vi "R1SBRControl_Status.vi"(7 "LabVIEW Web Service Request":refnum<class "Web Request.lvclass">) -> (0 "error out":errorcluster, 3 "SBRData":T1)   [LabVIEW 2016]
uses:
  <vilib>/wsapi/Web Request.lvclass
  R1Controls/R1SBR_Status.ctl
  R1Controls/R1SBR_SetParams.ctl
panel:
  # "Use the Web Service Request input terminal to call the VIs on the Web Services palette. Do not remove it from the connector pane unless you don't need access to the palette."
  # "Each additional control wired to the connector pane will be available as an input in the URL. To include an indicator in terminal-mode output (the default setting), it must also be wired to the connector pane."
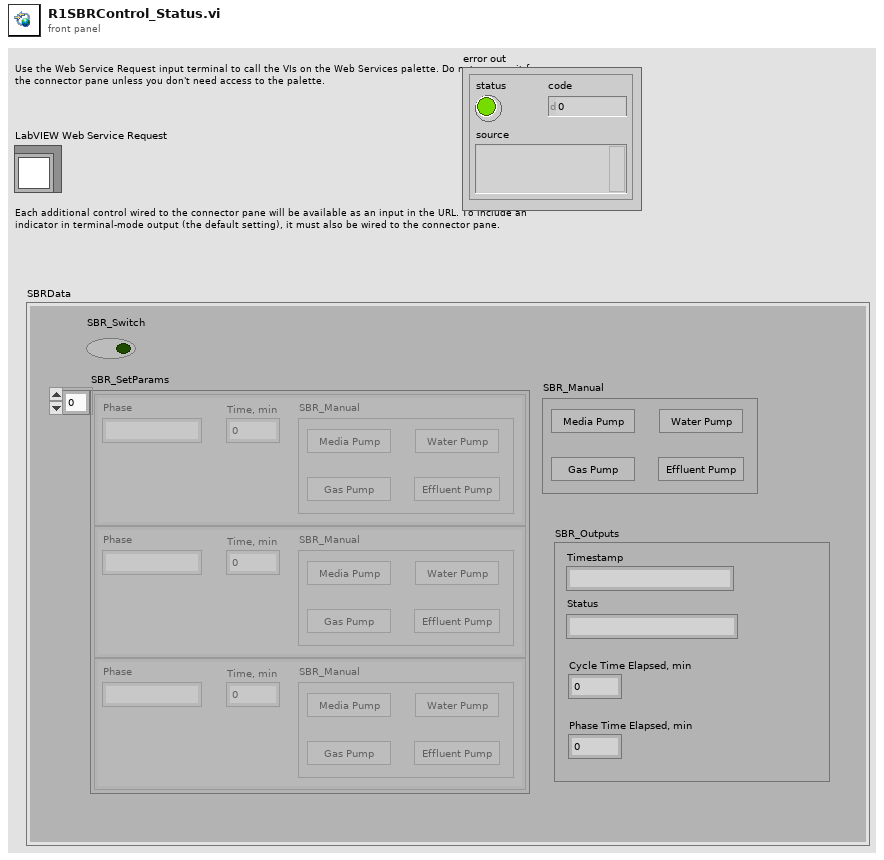
[diagram p1: front panel]
types:
  T1 = typedef "R1SBR_Status.ctl" = cluster{"SBR_Switch":bool, "SBR_SetParams":T2, "SBR_Manual":cluster{"Media Pump":bool, "Water Pump":bool, "Gas Pump":bool, "Effluent Pump":bool}, "SBR_Outputs":cluster{"Cycle Time Elapsed, min":dbl, "Phase Time Elapsed, min":dbl, "Timestamp":string, "Status":string}}
  T2 = typedef "R1SBR_SetParams.ctl" = cluster{"Phase":string, "Time, min":dbl, "SBR_Manual":cluster{"Media Pump":bool, "Water Pump":bool, "Gas Pump":bool, "Effluent Pump":bool}}[]
  T3 = cluster{"Media Pump":bool, "Water Pump":bool, "Gas Pump":bool, "Effluent Pump":bool}
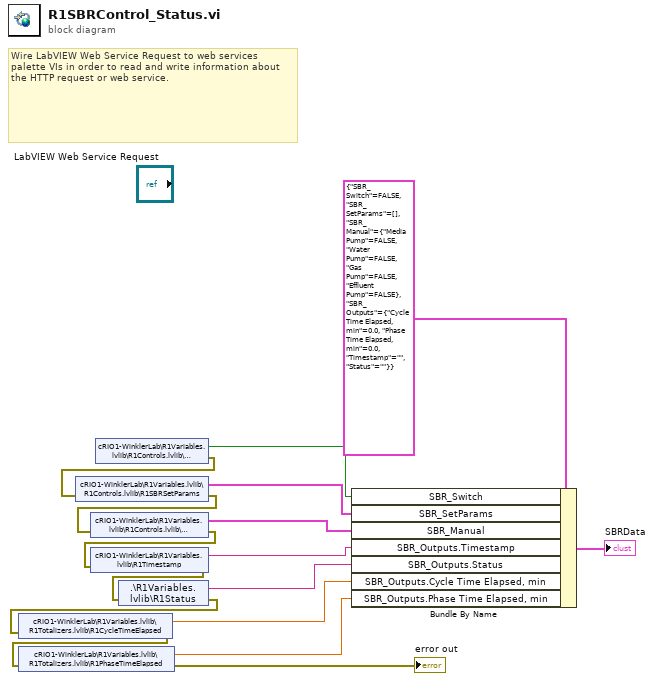
[diagram p0: block diagram]
diagram:
  # "Wire LabVIEW Web Service Request to web services palette VIs in order to read and write information about the HTTP request or web service."
  n1 = shared-variable "cRIO1-WinklerLab\\R1Variables.lvlib\\R1Controls.lvlib\\R1SBRSwitch"() -> (w14:bool, error out=w9:errorcluster)  [unwired: 1 in]
  n2 = shared-variable "cRIO1-WinklerLab\\R1Variables.lvlib\\R1Controls.lvlib\\R1SBRSetParams"(error in=w9) -> (w15:T2, error out=w8:errorcluster)
  n3 = shared-variable "cRIO1-WinklerLab\\R1Variables.lvlib\\R1Controls.lvlib\\R1SBRManual"(error in=w8) -> (w16:T3, error out=w7:errorcluster)
  n4 = shared-variable "cRIO1-WinklerLab\\R1Variables.lvlib\\R1Timestamp"(error in=w7) -> (w4:string, error out=w2:errorcluster)
  n5 = shared-variable ".\\R1Variables.lvlib\\R1Status"(error in=w2) -> (w3:string, error out=w6:errorcluster)
  n6 = shared-variable "cRIO1-WinklerLab\\R1Variables.lvlib\\R1Totalizers.lvlib\\R1CycleTimeElapsed"(error in=w6) -> (w13:dbl, error out=w1:errorcluster)
  n7 = shared-variable "cRIO1-WinklerLab\\R1Variables.lvlib\\R1Totalizers.lvlib\\R1PhaseTimeElapsed"(error in=w1) -> (w12:dbl, error out=→"error out":errorcluster)
  n8 = Bundle By Name(cluster=T1 {"SBR_Switch"=FALSE, "SBR_SetParams"=[], "SBR_Manual"={"Media Pump"=FALSE, "Water Pump"=FALSE, "Gas Pump"=FALSE, "Effluent Pump"=FALSE}, "SBR_Outputs"={"Cycle Time Elapsed, min"=0.0, "Phase Time Elapsed, min"=0.0, "Timestamp"="", "Status"=""}} ("SBRData"), "SBR_Switch"=w14, "SBR_SetParams"=w15, "SBR_Manual"=w16, "SBR_Outputs.Timestamp"=w4, "SBR_Outputs.Status"=w3, "SBR_Outputs.Cycle Time Elapsed, min"=w13, "SBR_Outputs.Phase Time Elapsed, min"=w12) -> (→"SBRData":T1)
